vi "mode_selection.vi"(5 "MeasSetId":i32) -> (0 "Coeff_selection":bool, 1 "String_selection":bool)   [LabVIEW 2016]
uses:
  TemperatureMeasure/Thermal_type.vi
panel:
  out "index_coeff":i32
  out "index_string":i32
  out "Tempcoeff":bool
  out "Tempstring":bool
  out "Length_string":i32
  out "Length_coeff":i32
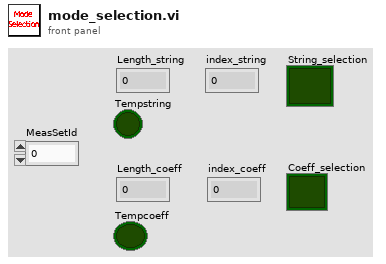
[diagram p1: front panel]
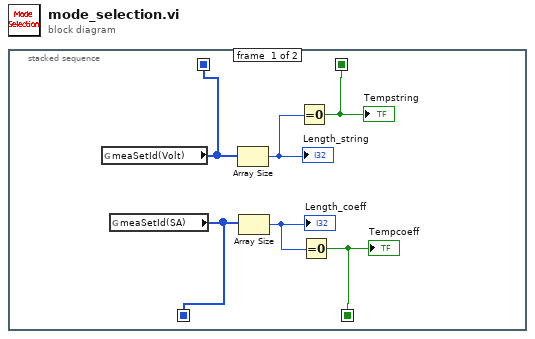
[diagram p0: block diagram]
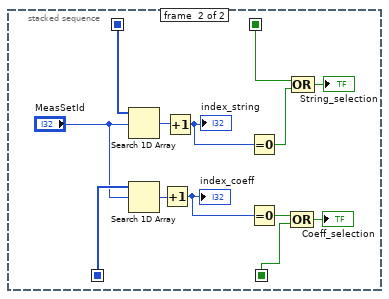
[diagram p2: hidden frame]
diagram:
  n1 = stacked-sequence {
    seq-local: [w4 _] -> [_ w19]
    seq-local: [w3 _] -> [_ w18]
    seq-local: [w2 _] -> [_ w14]
    seq-local: [w1 _] -> [_ w9]
    frame #0 {
      n2 = global read "Thermal_type.vi" "meaSetId(Volt)"() -> (w4:i32[])
      n3 = global read "Thermal_type.vi" "meaSetId(SA)"() -> (w3:i32[])
      n4 = Array Size(array=w4) -> (size(s)=w6:i32)
      "Length_string" <- w6
      n5 = Array Size(array=w3) -> (size(s)=w5:i32)
      "Length_coeff" <- w5
      n6 = Equal To 0?(x=w6) -> (x = 0?=w2:bool)
      "Tempstring" <- w2
      n7 = Equal To 0?(x=w5) -> (x = 0?=w1:bool)
      "Tempcoeff" <- w1
    }
    frame #1 {
      n8 = Search 1D Array(1D array=w19, element="MeasSetId") -> (index of element=w16:i32)  [unwired: 1 in]
      n9 = Search 1D Array(1D array=w18, element="MeasSetId") -> (index of element=w15:i32)  [unwired: 1 in]
      n10 = Increment(x=w15) -> (x+1=w10:i32)
      "index_coeff" <- w10
      n11 = Increment(x=w16) -> (x+1=w13:i32)
      "index_string" <- w13
      n12 = Equal To 0?(x=w13) -> (x = 0?=w12:bool)
      n13 = Equal To 0?(x=w10) -> (x = 0?=w11:bool)
      n14 = Compound Arithmetic op=OR(w11, w9) -> (→"Coeff_selection":bool)
      n15 = Compound Arithmetic op=OR(w14, w12) -> (→"String_selection":bool)
    }
  }
